vi "reql_response.vi"(8 "error in (no error)":errorcluster, 11 "response":string) -> (0 "error out":errorcluster, 3 "values":variant[](array[variant]), 4 "response":variant)   [LabVIEW 2017, in "rethinkdb.lvlib"]
uses:
  rethinkdb.lvlib
  914ac796-27b2-451e-b7e8-bb850beead6e.vi
  baeb6880-b455-45bd-8c2a-24346e5095c7.vi
  json_get_names.vi
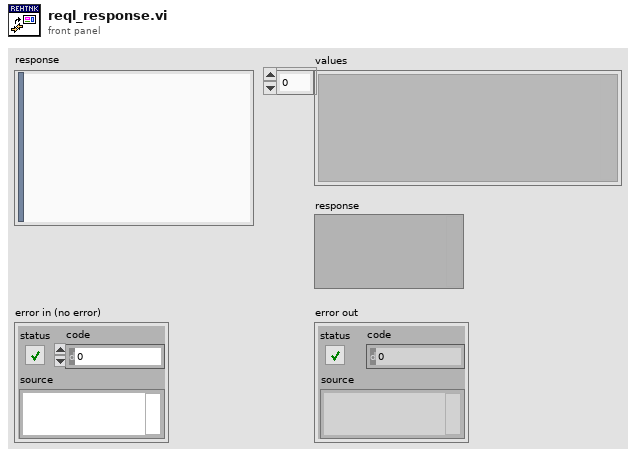
[diagram p1: front panel]
types:
  T1 = typedef "rethinkdb.lvlib/ql2_response.ctl" = enum8{"SUCCESS_ATOM", "SUCCESS_SEQUENCE", "SUCCESS_PARTIAL", "WAIT_COMPLETE", "SERVER_INFO", "CLIENT_ERROR", "COMPILE_ERROR", "RUNTIME_ERROR", "invalid"}
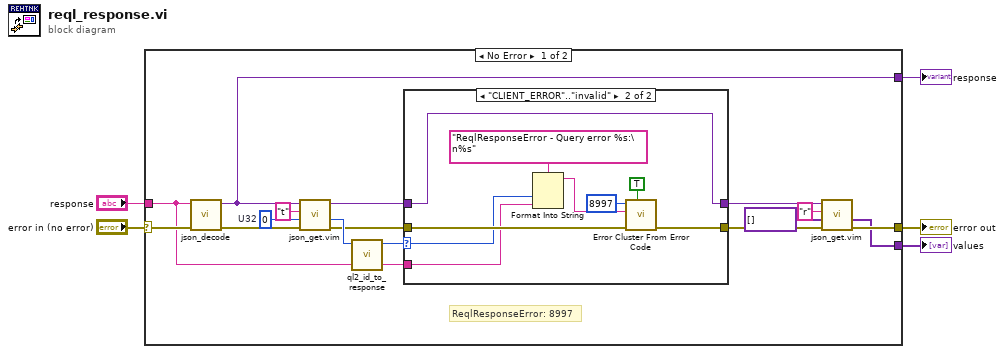
[diagram p0: block diagram]
diagram:
  n1 = case shown="No Error" "error in (no error)" {
    selector: "error in (no error)" -> [w21 w33]
    tunnel: [w11 w33] -> w4
    tunnel: "response" -> [w8 _]
    tunnel: [w7 _] -> w2
    tunnel: [w6 _] -> w1
    frame No Error {
      w18 = u32 0  # U32
      # "ReqlResponseError: 8997"
      n2 = call "json_decode.vi"("error in (no error)"=w21, "json"=w8) -> ("error out"=w20:errorcluster, "variant"=w6:variant)  [unwired: 8 in]
      n3 = call "json_get.vim"("error in (no error)"=w20, "default"=w18, "name"="t" ("key"), "variant in"=w6) -> ("error out"=w14:errorcluster, "value"=w17:u32, "variant out"=w15:variant)  [unwired: 4 in, 1 out]
      n4 = call "ql2_id_to_response.vi"("id"=w17) -> ("response_type"=w16:T1)  [unwired: 10 in]
      n5 = case shown="\"CLIENT_ERROR\"..\"invalid\"" w16 {
        selector: w16 -> [_ w25]
        tunnel: w15 -> [w22 w32]
        tunnel: w14 -> [w23 w27]
        tunnel: [w23 w26] -> w12
        tunnel: [w22 w32] -> w10
        tunnel: w8 -> [_ w24]
        frame "SUCCESS_ATOM".."SERVER_INFO" {
        }
        frame "CLIENT_ERROR".."invalid" {
          n6 = Format Into String(format string="ReqlResponseError - Query error %s:\n%s" ("error message (\"\")"), w25, w24) -> (resulting string=w31:string)  [unwired: 2 in, 1 out]
          n7 = call <vilib>:"Error Cluster From Error Code.vi"("show call chain? (False)"=TRUE, "error in (no error)"=w27, "error message (\"\")"=w31, "error code (0)"=8997) -> ("error out"=w26:errorcluster)  [unwired: 5 in]
        }
      }
      n8 = call "json_get.vim"("error in (no error)"=w12, "default"=variant[] [], "name"="r" ("key"), "variant in"=w10) -> ("error out"=w11:errorcluster, "value"=w7:variant[])  [unwired: 4 in, 2 out]
    }
    frame Error {
    }
  }
  "error out" <- w4
  "values" <- w2
  "response" <- w1
